vi "DPO_7K_MinValue_measurement.vi"(8 "Error In":errorcluster, 10 "Channel":u16(ring) items=["Channel 1", "Channel 2", "Channel 3", "Channel 4", "Math 1", "Math 2", "Math 3", "Math 4", "Reference 1", "Reference 2", "Reference 3", "Reference 4"], 11 "VISA resource name in":refnum<visa-resource-name>) -> (0 "Error Out":errorcluster, 2 "Min Value":dbl, 3 "VISA resource name out":refnum<visa-resource-name>)   [LabVIEW 2020]
uses:
  subVI/Set_Configuration.ctl
  subVI/Return_To_Interface.ctl
panel:
  in  "Return to Interface":T1
  in  "Set":T2
  # "MIN VALUE MEASUREMENT"
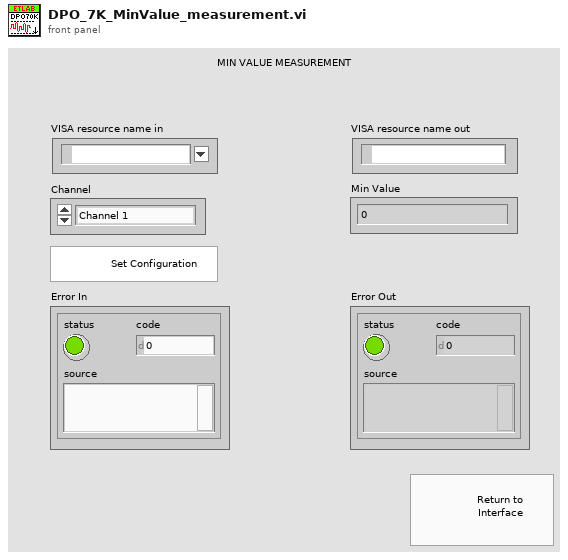
[diagram p1: front panel]
types:
  T1 = typedef "Return_To_Interface.ctl" = bool
  T2 = typedef "Set_Configuration.ctl" = bool
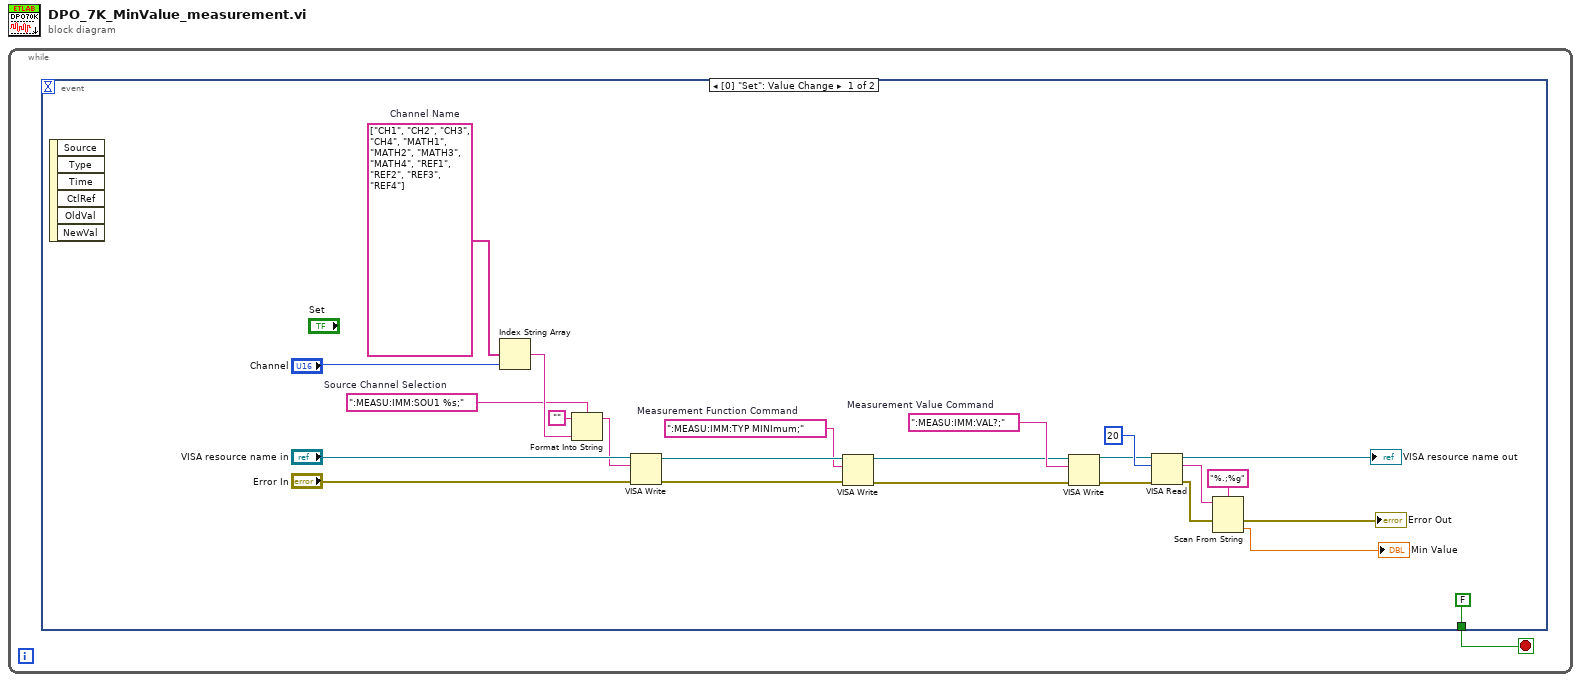
[diagram p0: block diagram]
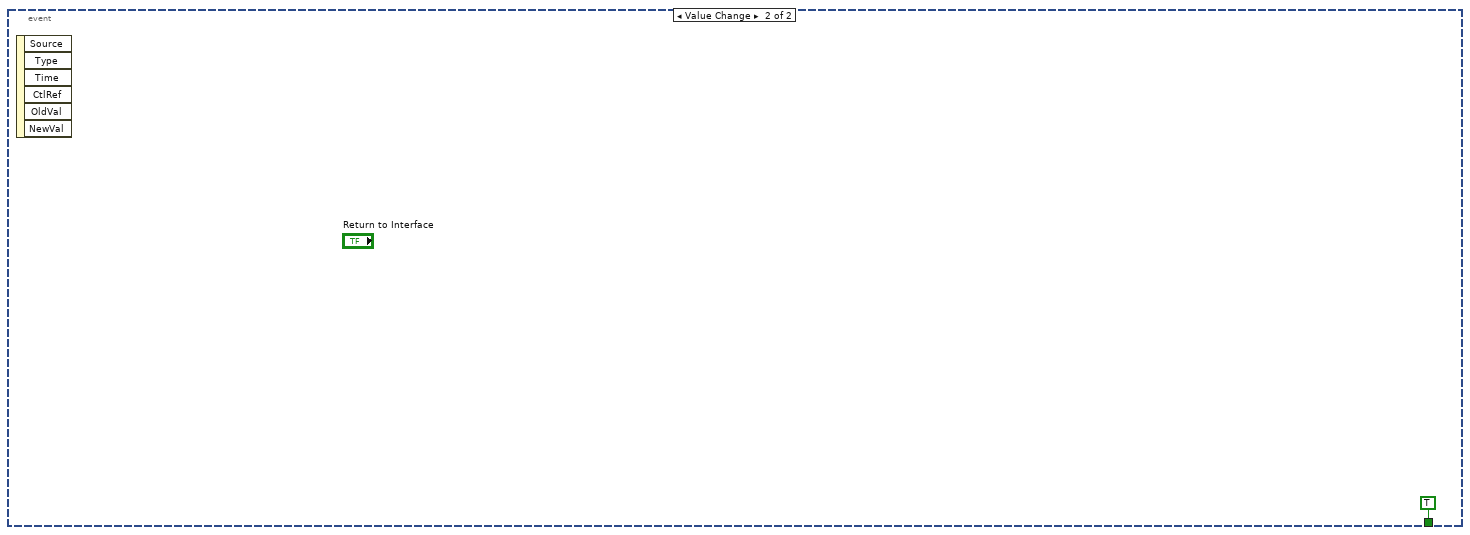
[diagram p2: hidden frame]
diagram:
  n1 = while {
    stop <- w1 stop-if-true
    n2 = event shown="[0] \"Set\": Value Change" {
      selector: _ -> [_ _]
      dyn-events: _ -> [_ _]
      timeout: _ -> [_ _]
      tunnel: [FALSE TRUE] -> w1
      event Value Change {
        w13 = ":MEASU:IMM:VAL?;"  # Measurement Value Command
        w14 = ":MEASU:IMM:TYP MINImum;"  # Measurement Function Command
        w20 = string[] ["CH1", "CH2", "CH3", "CH4", "MATH1", "MATH2", "MATH3", "MATH4", "REF1", "REF2", "REF3", "REF4"]  # Channel Name
        w21 = ":MEASU:IMM:SOU1 %s;"  # Source Channel Selection
        n3 = event-data() -> ()  [unwired: 1 in, 6 out]
        n4 = Index String Array(1:"Channel", 2:w20) -> (0:w22:string)  [unwired: 1 in]
        n5 = Format Into String(format string=w21, initial string="", w22) -> (resulting string=w18:string)  [unwired: 1 in, 1 out]
        n6 = VISA Write(VISA resource name="VISA resource name in", write buffer=w18, error in (no error)="Error In") -> (VISA resource name out=w16:refnum<visa-resource-name>, error out=w15:errorcluster)  [unwired: 1 out]
        n7 = VISA Write(VISA resource name=w16, write buffer=w14, error in (no error)=w15) -> (VISA resource name out=w12:refnum<visa-resource-name>, error out=w11:errorcluster)  [unwired: 1 out]
        n8 = VISA Write(VISA resource name=w12, write buffer=w13, error in (no error)=w11) -> (VISA resource name out=w6:refnum<visa-resource-name>, error out=w5:errorcluster)  [unwired: 1 out]
        n9 = VISA Read(VISA resource name=w6, byte count=u32 20, error in (no error)=w5) -> (VISA resource name out=→"VISA resource name out":refnum<visa-resource-name>, read buffer=w7:string, error out=w8:errorcluster)  [unwired: 1 out]
        n10 = Scan From String(format string="%.;%g", input string=w7, error in=w8) -> (error out=→"Error Out":errorcluster, output 1=→"Min Value":dbl)  [unwired: 2 in, 2 out]
      }
      event Value Change {
        n11 = event-data() -> ()  [unwired: 1 in, 6 out]
      }
    }
  }
